vi "GetPhysicalOutputChConfig.vi"(8 "error in (no error)":errorcluster, 11 "Highland T564 DDG in":refnum<class "Highland T564 DDG.lvclass">) -> (0 "error out":errorcluster, 3 "Highland T564 DDG out":refnum<class "Highland T564 DDG.lvclass">)   [LabVIEW 2020, in "Highland T564 DDG.lvclass"]
uses:
  Highland T564 DDG.lvclass
  C:/GEECS/Developers Version/source/Device Drivers/shared/MetaDriver_v1/MetaDriver_v1.lvclass
  Channel.ctl
  Choice83.ctl
  Choice01.ctl
  Choice84.ctl
  Highland T564 DDG.lvclass/Highland T564 DDG.ctl
  T560Session.lvclass
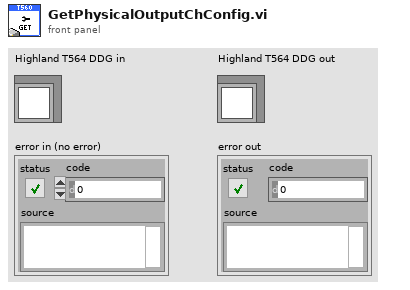
[diagram p1: front panel]
types:
  T1 = typedef "Channel.ctl" = cluster{"Polarity":T2, "ChannelOn":enum16{"off", "on"}, "Delay":T3, "Width":T3, "ChannelName":T4}
  T2 = typedef "Choice83.ctl" = enum16{"Direct", "Inverted"}
  T3 = typedef "Choice01.ctl" = cluster{"Value":dbl, "Min":dbl, "Max":dbl, "StepSize":dbl, "Tolerance":dbl, "ValueActual":dbl}
  T4 = typedef "Choice84.ctl" = enum16{"Null", "A", "B", "C", "D", "Trigger"}
  T5 = typedef "T560Channel.lvclass/ChannelName.ctl" = enum16{"Null", "A", "B", "C", "D", "Trigger"}
  T6 = cluster{"PropertiesAccess:ChannelOn":bool, "PropertiesAccess:Delay":string, "PropertiesAccess:Polarity":enum16{"Direct", "Inverted"}, "PropertiesAccess:Width":string, "ChannelName":T5}
  T7 = typedef "Highland T564 DDG.lvclass/settings Highland T560 DDG_TypDef.ctl" = cluster{"VisaResource":string, "BaudRate":u32, "Save":enum16{"off", "on"}, "LocalSavingPath":path, "Trigger":T8, "Channel1":T1, "Channel2":T1, "Channel3":T1, "Channel4":T1, "Simulation":T11}
  T8 = typedef "Trigger.ctl" = cluster{"Divisor":T3, "Level":T3, "Impedance":T9, "Source":T10}
  T9 = typedef "TriggerImpedance.ctl" = enum16{"10KOhm", "50Ohms"}
  T10 = typedef "TriggerSource.ctl" = enum16{"Rising", "Falling", "Internal 80MHz", "Internal DDS", "Remote", "Disabled"}
  T11 = typedef "OnOffTypeDef.ctl" = enum16{"off", "on"}
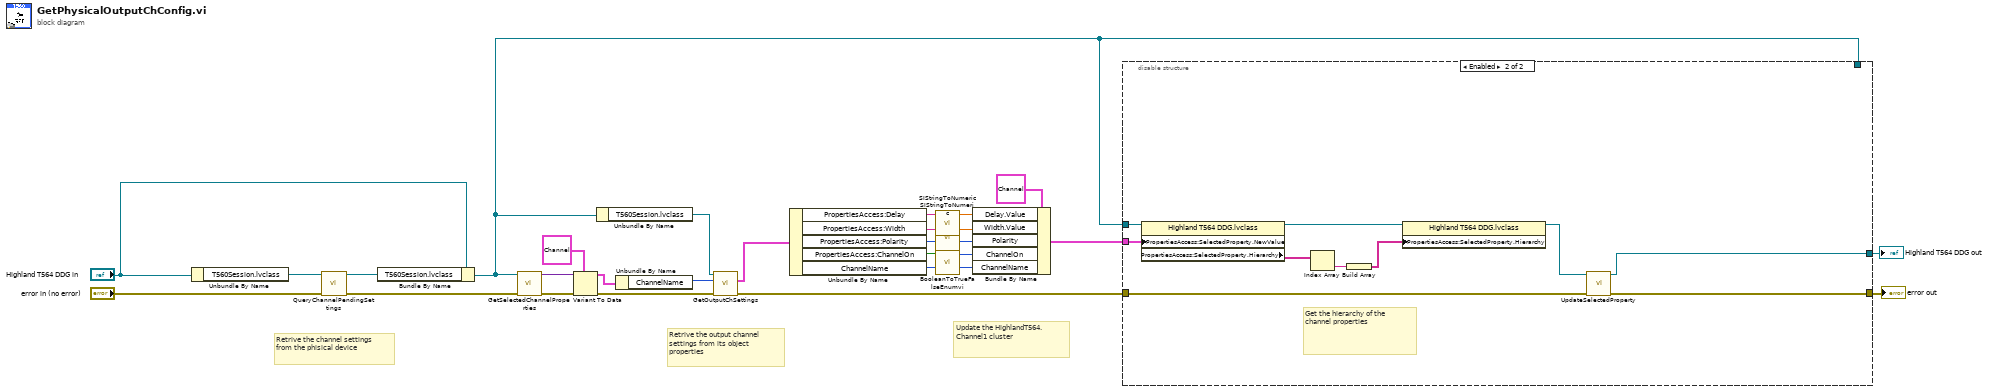
[diagram p0: block diagram]
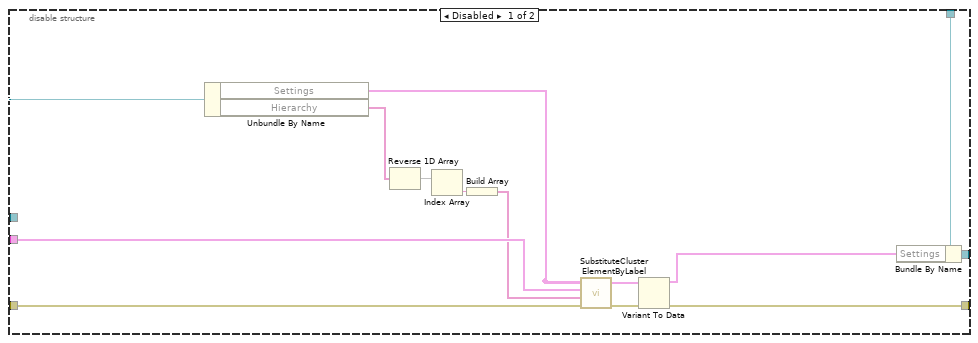
[diagram p2: hidden frame]
diagram:
  # "Update the HighlandT564.Channel1 cluster"
  # "Retrive the channel settings from the phisical device"
  # "Retrive the output channel settings from its object properties"
  n1 = Unbundle By Name("Highland T564 DDG in") -> ("T560Session.lvclass"=w27:refnum<class "T560Session.lvclass">)
  n2 = call-dynamic "QueryChannelPendingSettings.vi"("error in"="error in (no error)", "T560Session in"=w27) -> ("error out"=w17:errorcluster, "T560Session out"=w13:refnum<class "T560Session.lvclass">)  [unwired: 8 in]
  n3 = Bundle By Name(cluster="Highland T564 DDG in", "T560Session.lvclass"=w13) -> (w1:refnum<class "Highland T564 DDG.lvclass">)
  n4 = call "GetSelectedChannelProperties.vi"("error in (no error)"=w17, "Highland T564 DDG in"=w1) -> ("error out"=w20:errorcluster, "ChannelProperties"=w19:variant)  [unwired: 8 in]
  n5 = Variant To Data(error in=w20, type=T1 {"Polarity"=enum."Direct", "ChannelOn"=enum."off", "Delay"={"Value"=0.0, "Min"=0.0, "Max"=0.0, "StepSize"=0.0, "Tolerance"=0.0, "ValueActual"=0.0}, "Width"={"Value"=0.0, "Min"=0.0, "Max"=0.0, "StepSize"=0.0, "Tolerance"=0.0, "ValueActual"=0.0}, "ChannelName"=enum."Null"} ("Settings.Channel1"), Variant=w19) -> (data=w18:T1, error out=w16:errorcluster)
  n6 = Unbundle By Name(w1) -> ("T560Session.lvclass"=w11:refnum<class "T560Session.lvclass">)
  n7 = Unbundle By Name(w18) -> ("ChannelName"=w15:T4)
  n8 = call-dynamic "GetOutputChSettings.vi"("error in (no error)"=w16, "ChannelName"=w15, "T560Session in"=w11) -> ("error out"=w10:errorcluster, "OutputSettings"=w12:T6)  [unwired: 6 in, 1 out]
  n9 = Unbundle By Name(w12) -> ("PropertiesAccess:Delay"=w25:string, "PropertiesAccess:Width"=w23:string, "PropertiesAccess:Polarity"=w6:enum16{"Direct", "Inverted"}, "PropertiesAccess:ChannelOn"=w4:bool, "ChannelName"=w5:T5)
  n10 = call "SIStringToNumeric.vi"("SI number"=w25) -> ("Number"=w24:dbl)  [unwired: 9 in, 1 out]
  n11 = call "SIStringToNumeric.vi"("SI number"=w23) -> ("Number"=w22:dbl)  [unwired: 9 in, 1 out]
  n12 = call "BooleanToTrueFalseEnumvi.vi"("selection"=w4) -> ("On/Off"=w3:enum16{"off", "on"})  [unwired: 10 in]
  n13 = Bundle By Name(cluster=T1 {"Polarity"=enum."Direct", "ChannelOn"=enum."off", "Delay"={"Value"=0.0, "Min"=0.0, "Max"=0.0, "StepSize"=0.0, "Tolerance"=0.0, "ValueActual"=0.0}, "Width"={"Value"=0.0, "Min"=0.0, "Max"=0.0, "StepSize"=0.0, "Tolerance"=0.0, "ValueActual"=0.0}, "ChannelName"=enum."Null"} ("Channel1"), "Delay.Value"=w24, "Width.Value"=w22, "Polarity"=w6, "ChannelOn"=w3, "ChannelName"=w5) -> (w2:T1)
  n14 = disable-structure shown="Enabled" {
    disable-tunnel: w10 -> [w40 w48]
    disable-tunnel: [w38 w46] -> w9
    disable-tunnel: [w37 w47] -> w8
    disable-tunnel: w2 -> [w36 w49]
    disable-tunnel: w1 -> [w35 _]
    disable-tunnel: w1 -> [_ w45]
    frame Disabled {
      n15 = Unbundle By Name(w35) -> ("Settings"=w33:T7, "Hierarchy"=w31:string[])
      n16 = Reverse 1D Array(array=w31) -> (reversed array=w30:string[])
      n17 = Index Array(array=w30) -> (element=w29:string)  [unwired: 1 in]
      n18 = Build Array(w29) -> (w28:string[])
      n19 = call "SubstituteClusterElementByLabel.vi"("error in (no error)"=w40, "ElementHierarchy"=w28, "NewElementValue"=w36, "ClusterIn"=w33) -> ("ErrorOut"=w34:errorcluster, "UpdatedClusterOut"=w32:variant)  [unwired: 5 in, 1 out]
      n20 = Variant To Data(error in=w34, type=w33, Variant=w32) -> (data=w39:T7, error out=w37:errorcluster)
      n21 = Bundle By Name(cluster=w35, "Settings"=w39) -> (w38:refnum<class "Highland T564 DDG.lvclass">)
    }
    frame Enabled {
      # "Get the hierarchy of the channel properties"
      n22 = property class="Highland T564 DDG.lvclass"(reference=w45, "PropertiesAccess:SelectedProperty.NewValue"=w49) -> (reference out=w50:refnum<class "Highland T564 DDG.lvclass">, "PropertiesAccess:SelectedProperty.Hierarchy"=w43:string[])  [unwired: 1 in, 1 out]
      n23 = Index Array(array=w43) -> (element=w42:string)  [unwired: 1 in]
      n24 = Build Array(w42) -> (w41:string[])
      n25 = property class="Highland T564 DDG.lvclass"(reference=w50, "PropertiesAccess:SelectedProperty.Hierarchy"=w41) -> (reference out=w44:refnum<class "Highland T564 DDG.lvclass">)  [unwired: 1 in, 1 out]
      n26 = call-dynamic "UpdateSelectedProperty.vi"("error in (no error)"=w48, "Highland T564 DDG in"=w44) -> ("error out"=w47:errorcluster, "Highland T564 DDG out"=w46:refnum<class "Highland T564 DDG.lvclass">)  [unwired: 8 in]
    }
  }
  "Highland T564 DDG out" <- w9
  "error out" <- w8
